vi "Write Key.vi"(8 "error in (no error)":errorcluster, 10 "Key":string, 11 "Update Setting in":refnum<class "Update Setting.lvclass">) -> (0 "error out":errorcluster, 3 "Update Setting out":refnum<class "Update Setting.lvclass">)   [LabVIEW 2014, in "Update Setting.lvclass"]
uses:
  Update Setting.lvclass
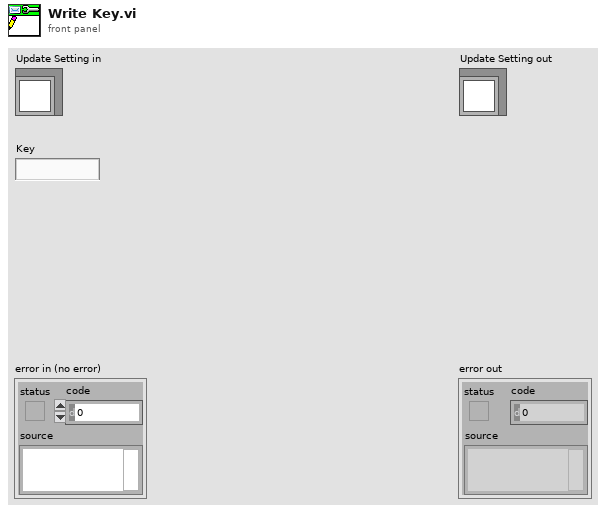
[diagram p1: front panel]
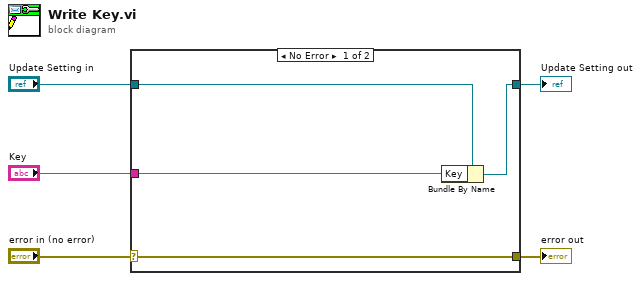
[diagram p0: block diagram]
diagram:
  n1 = case shown="No Error" "error in (no error)" {
    selector: "error in (no error)" -> [w9 w10]
    tunnel: [w9 w10] -> w4
    tunnel: [w7 w11] -> w2
    tunnel: "Update Setting in" -> [w8 w11]
    tunnel: "Key" -> [w6 _]
    frame No Error {
      n2 = Bundle By Name(cluster=w8, "Key"=w6) -> (w7:refnum<class "Update Setting.lvclass">)
    }
    frame Error {
    }
  }
  "error out" <- w4
  "Update Setting out" <- w2
